vi "gandlionread.vi"() -> ()   [LabVIEW 2024]
panel:
  out "String":string
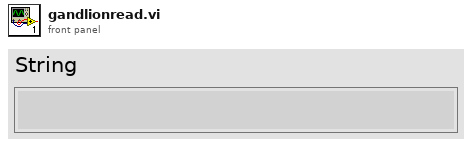
[diagram p1: front panel]
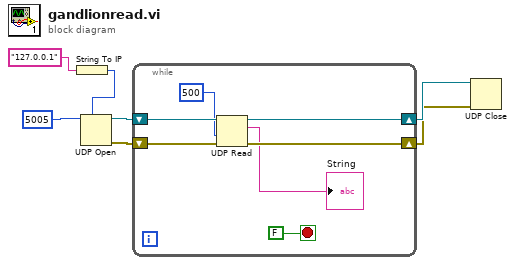
[diagram p0: block diagram]
diagram:
  n1 = String To IP(1:"127.0.0.1") -> (0:w1:u32)
  n2 = UDP Open(7:w1, 11:u16 5005 ("port")) -> (port=w6:refnum<k16>, 0:w4:errorcluster)  [unwired: 3 in, 1 out]
  n3 = while {
    shift-right: [w13] -> w5
    shift-left: w6 -> [w14]
    shift-right: [w11] -> w3
    shift-left: w4 -> [w12]
    stop <- FALSE stop-if-true
    n4 = UDP Read(connection ID=w14, timeout ms (25000)=500, 8:w12) -> (data out=→"String":string, error out=w11:errorcluster, 3:w13:refnum<k16>)  [unwired: 1 in, 2 out]
  }
  n5 = UDP Close(connection ID=w5, 8:w3) -> ()  [unwired: 2 out]
